vi "Random pump waveplate tester.vi"() -> ()   [LabVIEW 2013]
panel:
  in  "Array":dbl[](array[numeric])
  out "64bit integer":i64
  in  "appended array":dbl[][](array[numeric])
  out "error out":errorcluster
  out "WP Error":bool=TRUE
  out "Current position (units)":dbl
  out "VISA Refnum out":refnum<visa-resource-name>
  in  "Trigger rate warnings?":bool
  in  "Trigger rate \nat 76 degrees":dbl
  in  "error in (no error)":errorcluster
  in  "Target trial \nlength (ms)":dbl
  in  "VISA Refnum in":refnum<visa-resource-name>
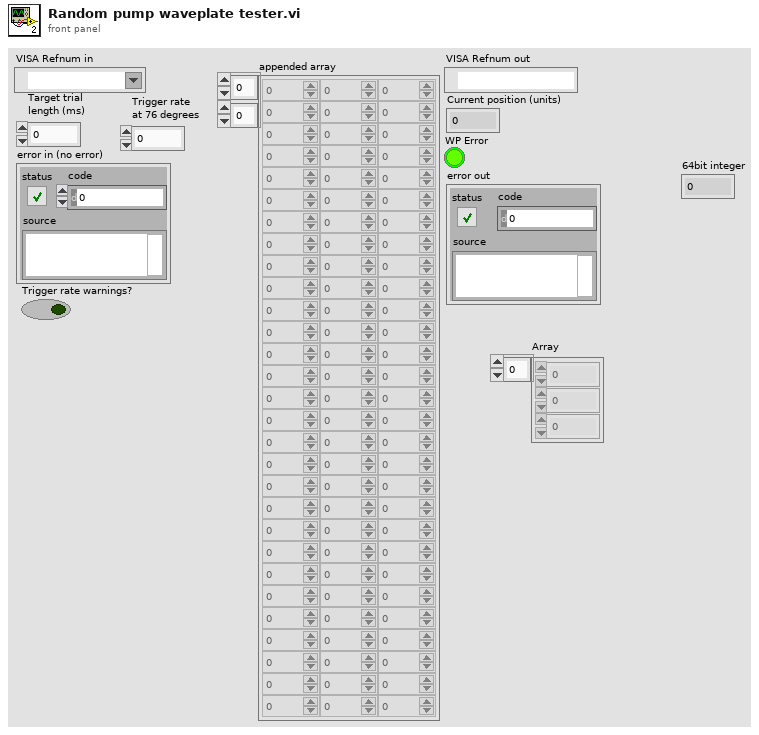
[diagram p1: front panel]
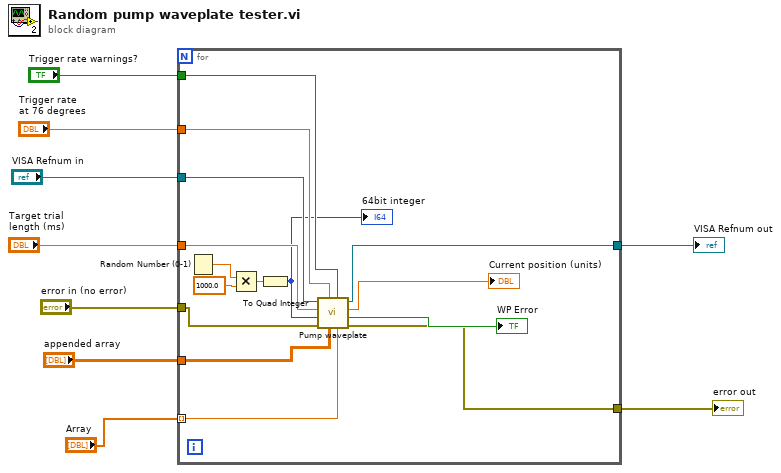
[diagram p0: block diagram]
diagram:
  n1 = for {
    tunnel: "VISA Refnum in" -> [w24]
    tunnel: "Target trial \nlength (ms)" -> [w23]
    tunnel: "error in (no error)" -> [w22]
    tunnel: "Trigger rate \nat 76 degrees" -> [w21]
    tunnel: "Trigger rate warnings?" -> [w20]
    tunnel: [w19] -> w4
    tunnel: [w16] -> w3
    tunnel: "appended array" -> [w15]
    tunnel: "Array" -> [w10] mode=indexing
    n2 = Random Number (0-1)() -> (number: 0 to 1=w14:dbl)
    n3 = Multiply(x=w14, y=1000.0) -> (x*y=w12:dbl)
    n4 = To Quad Integer(1:w12) -> (0:w11:i64)
    "64bit integer" <- w11
    n5 = call "Pump waveplate.vi"("Axis in"=w10, "Trigger rate warnings?"=w20, "appended array"=w15, "Trigger rate \nat 76 degrees"=w21, "error in (no error)"=w22, "Photon #"=w11, "Target trial \nlength (ms)"=w23, "VISA Refnum in"=w24) -> ("error out"=w16:errorcluster, "WP Error"=→"WP Error":bool, "Current position (units)"=→"Current position (units)":dbl, "VISA Refnum out"=w19:refnum<visa-resource-name>)
  }
  "VISA Refnum out" <- w4
  "error out" <- w3
